vi "Nano_Monitor.vi"() -> ()   [LabVIEW 2012]
uses:
  <vilib>/measure/NI_MABase.lvlib
  Madlib.dll
panel:
  in  "Axis":u32
  in  "signal type":T1(ring)
  in  "Amplitude (um)":dbl=10.0 min=0.0 max=100.0 step=0.5 format="%.3f"
  in  "X Control um":dbl(knob)=50.0 min=0.0 max=100.0 step=1.0 scale=0.0..100.0 scale format="%.3f"
  out "X Position um":dbl(graph)
  in  "?":bool
  # "X = 1\nY = 2\nZ = 3"
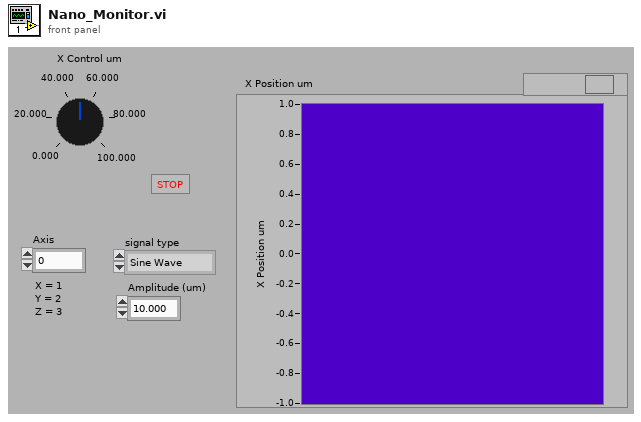
[diagram p1: front panel]
types:
  T1 = enum16{"Sine Wave", "Triangle Wave", "Square Wave", "Sawtooth Wave"}
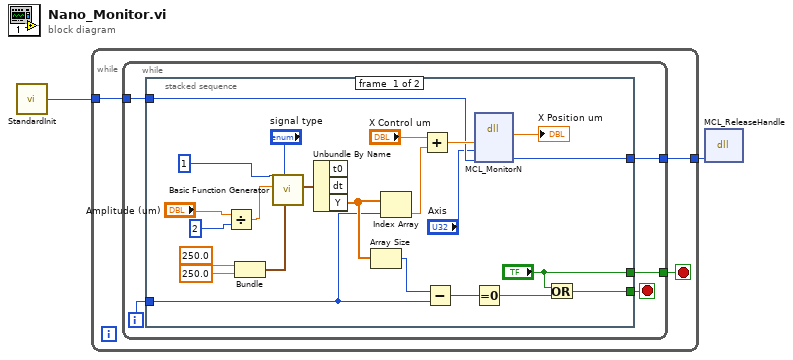
[diagram p0: block diagram]
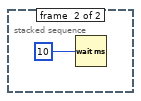
[diagram p2: hidden frame]
diagram:
  n1 = call "StandardInit.vi"() -> ("Outgoing Handle"=w1:i32)  [unwired: 1 in]
  n2 = while {
    tunnel: w1 -> [w4]
    tunnel: [w3] -> w2
    stop <- w5 stop-if-true
    n3 = while {
      tunnel: [w10] -> w5
      tunnel: w4 -> [w9]
      tunnel: [w8] -> w3
      i -> [w7]
      stop <- w6 stop-if-true
      n4 = stacked-sequence {
        tunnel: ["?" _] -> w10
        tunnel: w9 -> [w16 _]
        tunnel: [w15 _] -> w8
        tunnel: w7 -> [w13 _]
        tunnel: [w12 _] -> w6
        frame #0 {
          n5 = Divide(x="Amplitude (um)", y=2) -> (x/y=w24:dbl)
          n6 = Bundle(250.0, 250.0) -> (w17:cluster{dbl, dbl})  [unwired: 1 in]
          n7 = call <vilib>:"Basic Function Generator.vi"("sampling info"=w17, "signal type"="signal type", "amplitude"=w24, "frequency"=1) -> ("signal out"=w31:waveform(dbl))  [unwired: 5 in, 2 out]
          n8 = Unbundle By Name(w31) -> ("Y"=w30:dbl[])  [unwired: 2 out]
          n9 = Array Size(array=w30) -> (size(s)=w29:i32)
          n10 = Index Array(array=w30, index=w13) -> (element=w32:dbl)
          n11 = Add(x="X Control um", y=w32) -> (x+y=w21:dbl)
          n12 = Subtract(x=w29, y=w13) -> (x-y=w28:i32)
          n13 = Equal To 0?(x=w28) -> (x = 0?=w27:bool)
          n14 = dll-call lib="C:/Users/Labview/Desktop/SRR/Madlib_x64/Labview Examples/MADLib.dll" fn="MCL_MonitorN" label="MonitorN"("position"=w21, "axis"="Axis", "handle"=w16) -> (→"X Position um":dbl, "handle"=w15:i32)  [unwired: 5 in, 2 out]
          n15 = Or(x="?", y=w27) -> (x .or. y?=w12:bool)
        }
        frame #1 {
          n16 = Wait (ms)(milliseconds to wait=10) -> ()  [unwired: 1 out]
        }
      }
    }
  }
  n17 = dll-call lib="C:/Users/Labview/Desktop/SRR/Madlib_x64/Labview Examples/MADLib.dll" fn="MCL_ReleaseHandle"("handle"=w2) -> ()  [unwired: 5 in, 2 out]
